vi "THERM2dll.vi"(8 "error in (no error)":errorcluster, 11 "Input Cluster":cluster{"t":dbl, "D":dbl, "z":dbl[]}={"t"=0.0, "D"=0.0, "z"=[0.0, 0.0, 0.0, 0.0, 0.0, 0.0, 0.0, 0.0, 0.0, 0.0, 0.0, 0.0, 0.0, 0.0, 0.0, 0.0, 0.0, 0.0, 0.0, 0.0]}) -> (0 "error out":errorcluster, 3 "Output Cluster":T1)   [LabVIEW 2021]
doc: "subroutine THERM2dll(t, d, z, p, e, h, s, cv, cp, w, zz, hjt, a, g, xkappa, beta, dpdd, d2pdd2, dpdt, dddt, dddp, d2pdt2, d2pdtd, d2udt2, spare)\n\nCompute thermal quantities as a function of temperature, density,\nand compositions using core functions (Helmholtz free energy, ideal\ngas heat capacity and various derivatives and integrals)\n\nThis routine is the same as THERM, except that additional properties are calculated.\n\nINPUTS:\n t--temperature [K]\n D--molar density [mol/L]\n z--composition [array of mol frac]\n\nOUTPUTS:\n p--pressure [kPa]\n e--internal energy [J/mol]\n h--enthalpy [J/mol]\n s--entropy [J/mol-K]\n Cv--isochoric heat capacity [J/mol-K]\n Cp--isobaric heat capacity [J/mol-K]\n w--speed of sound [m/s]\n zz--compressibility factor (= PV/RT) [dimensionless]\n hjt--isenthalpic Joule-Thomson coefficient [K/kPa]\n a--Helmholtz energy [J/mol]\n g--Gibbs free energy [J/mol]\n xkappa--isothermal compressibility (= -1/V dV/dP = 1/rho dD/dP) [1/kPa]\n beta--volume expansivity (= 1/V dV/dT = -1/rho dD/dT) [1/K]\n dpdd--derivative dP/drho [kPa-L/mol]\n d2pdd2--derivative d^2P/drho^2 [kPa-L^2/mol^2]\n dpdt--derivative dP/dT [kPa/K]\n dddt--derivative drho/dT [mol/(L-K)]\n dddp--derivative drho/dP [mol/(L-kPa)]\n d2pdt2--derivative d2P/dT2 [kPa/K^2]\n d2pdtd--derivative d2P/dTd(rho) [J/mol-K]\n d2udt2--J/mol/k^2\n spare-- space holders for possible future properties"
uses:
  REFPROP.dll
panel:
  # "REFPROP-THERM2dll.vi"
  # "void THERM2dll(double *t, double *D, double *z, double *p, double *e, double *h, double *s, double *Cv, double *Cp, double *w, double *zz, double *hjt, double *a, double *g, double *xkappa, double *beta, double *dpdd, double *d2pdd2, double *dpdt, double *dddt, double *dddp, double *d2pdt2, double *d2pdtd, double *d2udt2, double *spare)"
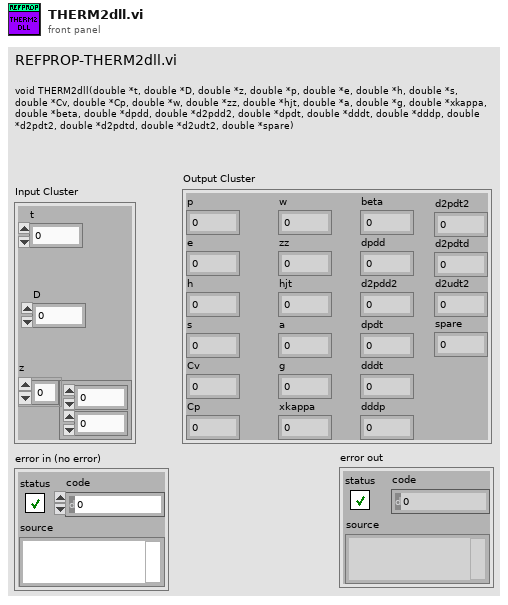
[diagram p1: front panel]
types:
  T1 = cluster{"p":dbl, "e":dbl, "h":dbl, "s":dbl, "Cv":dbl, "Cp":dbl, "w":dbl, "zz":dbl, "hjt":dbl, "a":dbl, "g":dbl, "xkappa":dbl, "beta":dbl, "dpdd":dbl, "d2pdd2":dbl, "dpdt":dbl, "dddt":dbl, "dddp":dbl, "d2pdt2":dbl, "d2pdtd":dbl, "d2udt2":dbl, "spare":dbl}
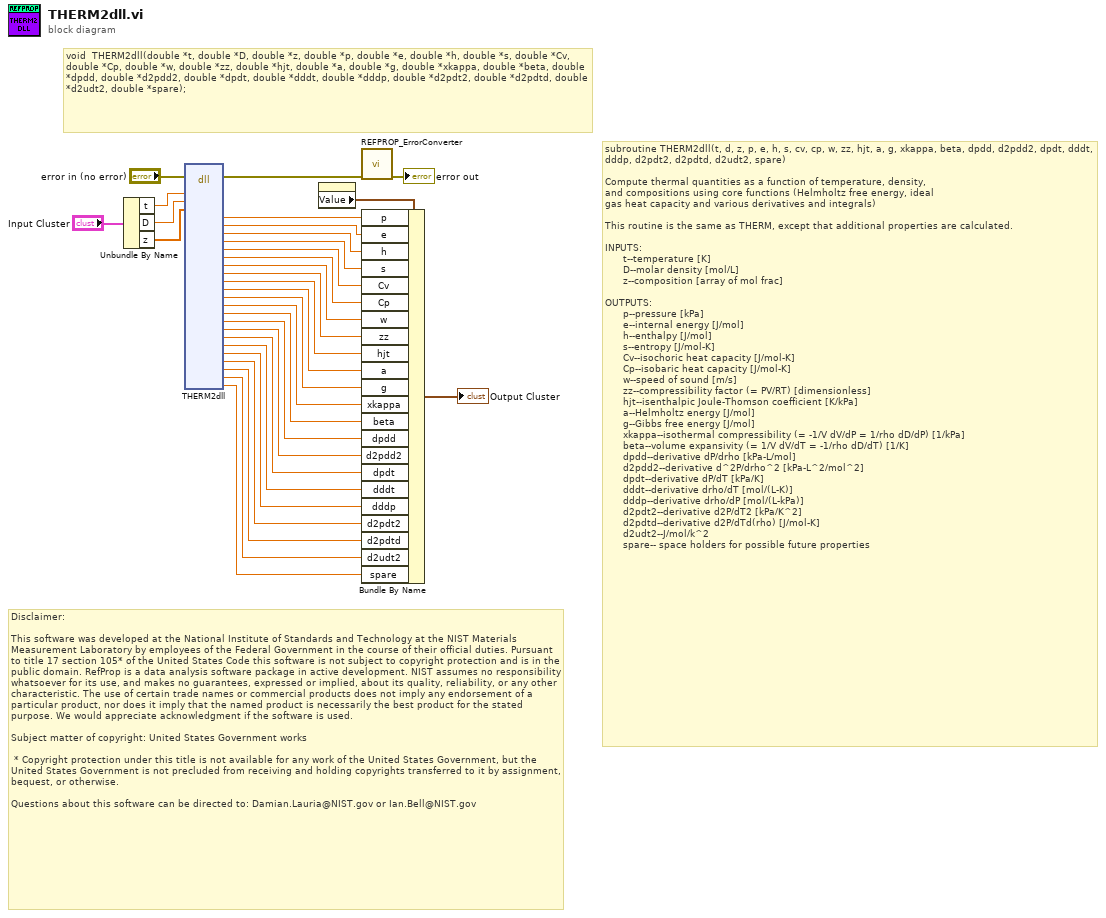
[diagram p0: block diagram]
diagram:
  # "Disclaimer:\n\nThis software was developed at the National Institute of Standards and Technology at the NIST Materials Measurement Laboratory by employees of the Federal Government in the course of their official duties. Pursuant to title 17 section 105* of the United States Code this software is not subject to copyright protection and is in the public domain. RefProp is a data analysis software package in active development. NIST assumes no responsibility whatsoever for its use, and makes no guarantees, expressed or implied, about its quality, reliability, or any other characteristic. The use of certain trade names or commercial products does not imply any endorsement of a particular product, nor does it imply that the named product is necessarily the best product for the stated purpose. We would appreciate acknowledgment if the software is used.\n \nSubject matter of copyright: United States Government works\n  \n * Copyright protection under this title is not available for any work of the United States Government, but the United States Government is not precluded from receiving and holding copyrights transferred to it by assignment, bequest, or otherwise.\n\nQuestions about this software can be directed to: Damian.Lauria@NIST.gov or Ian.Bell@NIST.gov"
  # "void  THERM2dll(double *t, double *D, double *z, double *p, double *e, double *h, double *s, double *Cv, double *Cp, double *w, double *zz, double *hjt, double *a, double *g, double *xkappa, double *beta, double *dpdd, double *d2pdd2, double *dpdt, double *dddt, double *dddp, double *d2pdt2, double *d2pdtd, double *d2udt2, double *spare);"
  # "subroutine THERM2dll(t, d, z, p, e, h, s, cv, cp, w, zz, hjt, a, g, xkappa, beta, dpdd, d2pdd2, dpdt, dddt, dddp, d2pdt2, d2pdtd, d2udt2, spare)\n\nCompute thermal quantities as a function of temperature, density,\nand compositions using core functions (Helmholtz free energy, ideal\ngas heat capacity and various derivatives and integrals)\n\nThis routine is the same as THERM, except that additional properties are calculated.\n\nINPUTS:\n      t--temperature [K]\n      D--molar density [mol/L]\n      z--composition [array of mol frac]\n\nOUTPUTS:\n      p--pressure [kPa]\n      e--internal energy [J/mol]\n      h--enthalpy [J/mol]\n      s--entropy [J/mol-K]\n      Cv--isochoric heat capacity [J/mol-K]\n      Cp--isobaric heat capacity [J/mol-K]\n      w--speed of sound [m/s]\n      zz--compressibility factor (= PV/RT) [dimensionless]\n      hjt--isenthalpic Joule-Thomson coefficient [K/kPa]\n      a--Helmholtz energy [J/mol]\n      g--Gibbs free energy [J/mol]\n      xkappa--isothermal compressibility (= -1/V dV/dP = 1/rho dD/dP) [1/kPa]\n      beta--volume expansivity (= 1/V dV/dT = -1/rho dD/dT) [1/K]\n      dpdd--derivative dP/drho [kPa-L/mol]\n      d2pdd2--derivative d^2P/drho^2 [kPa-L^2/mol^2]\n      dpdt--derivative dP/dT [kPa/K]\n      dddt--derivative drho/dT [mol/(L-K)]\n      dddp--derivative drho/dP [mol/(L-kPa)]\n      d2pdt2--derivative d2P/dT2 [kPa/K^2]\n      d2pdtd--derivative d2P/dTd(rho) [J/mol-K]\n      d2udt2--J/mol/k^2\n      spare-- space holders for possible future properties"
  n1 = Unbundle By Name("Input Cluster") -> ("t"=w30:dbl, "D"=w29:dbl, "z"=w28:dbl[])
  n2 = dll-call lib="C:/Users/lauria/OneDrive - National Institute of Standards and Technology (NIST)/LabVIEW Projects/7 REFPROP/REFPROP-wrappers-master/REFPROP-wrappers-master/wrappers/Labview/REFPROP/REFPROP.*" fn="THERM2dll"(error in="error in (no error)", "t"=w30, "D"=w29, "z"=w28) -> (error out=w31:errorcluster, "p"=w23:dbl, "e"=w22:dbl, "h"=w21:dbl, "s"=w20:dbl, "Cv"=w19:dbl, "Cp"=w18:dbl, "w"=w17:dbl, "zz"=w16:dbl, "hjt"=w15:dbl, "a"=w14:dbl, "g"=w13:dbl, "xkappa"=w12:dbl, "beta"=w11:dbl, "dpdd"=w10:dbl, "d2pdd2"=w9:dbl, "dpdt"=w8:dbl, "dddt"=w7:dbl, "dddp"=w6:dbl, "d2pdt2"=w5:dbl, "d2pdtd"=w4:dbl, "d2udt2"=w3:dbl, "spare"=w2:dbl)  [unwired: 28 in, 1 out]
  n3 = property on="Output Cluster" class="Clust (strict)"() -> ("Value"=w24:T1)  [unwired: 2 in, 2 out]
  n4 = call "REFPROP_ErrorConverter.vi"("error in (no error)"=w31) -> ("error out"=→"error out":errorcluster)  [unwired: 10 in]
  n5 = Bundle By Name(cluster=w24, "p"=w23, "e"=w22, "h"=w21, "s"=w20, "Cv"=w19, "Cp"=w18, "w"=w17, "zz"=w16, "hjt"=w15, "a"=w14, "g"=w13, "xkappa"=w12, "beta"=w11, "dpdd"=w10, "d2pdd2"=w9, "dpdt"=w8, "dddt"=w7, "dddp"=w6, "d2pdt2"=w5, "d2pdtd"=w4, "d2udt2"=w3, "spare"=w2) -> (→"Output Cluster":T1)
